vi "Get Ring Items.vi"(8 "error in (no error)":errorcluster, 11 "Scan Driver in":refnum<class "Scan Driver.lvclass">) -> (0 "error out":errorcluster, 1 "Reader":T2=enum."Photon Counter", 2 "Scanner":T1=enum."Magnetic Field", 3 "Scan Driver out":refnum<class "Scan Driver.lvclass">)   [LabVIEW 2012, in "Scan Driver.lvclass"]
doc: "If the object contains an \"XYZ.lvclass\", return the ring value for \"XYZ\". Class names must match the ring items exactly!"
uses:
  Scan Driver.lvclass
  Reader List.ctl
  Scanner List.ctl
  Scan Driver.lvclass/Scan Driver.ctl
  Readers/Reader/Reader.lvclass
panel:
  out "Reader name":string
  out "Scanner name":string
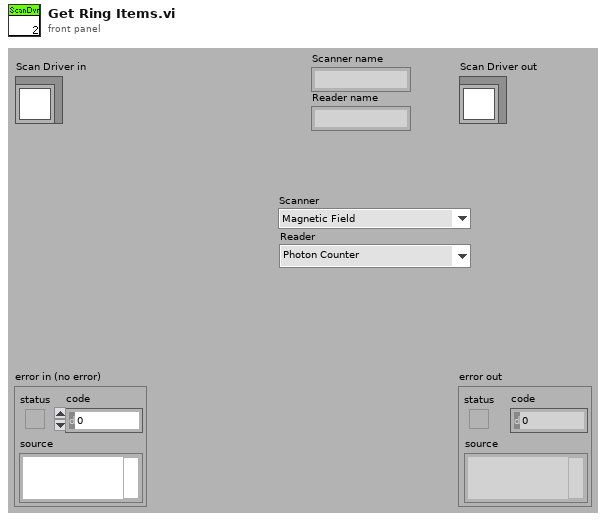
[diagram p1: front panel]
types:
  T1 = typedef "Scan Driver.lvclass/Scanner List.ctl" = enum16{"Analog Output Scan", "Continuous", "Dummy Scan", "Function Gen Scan", "Magnetic Field", "Magna Current Scan", "Magna Voltage Scan", "Microwave Freq Scan", "Pulse Gen Scan", "Pulse Gen Basic Scan", "Translation Stage Dual", "Wavelength", "Wavelength Digikröm", "Wavelength ActiveX", "Translation Stage Coarse", "Translation Stage Fine", "None"}
  T2 = typedef "Scan Driver.lvclass/Reader List.ctl" = enum16{"Anritsu Power Meter", "DAQmx Analog", "Dummy", "Lockin SR830", "Multimeter", "Photon Counter", "Power Meter", "Temperature Control"}
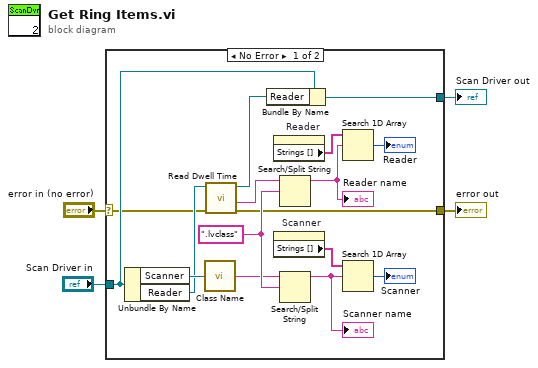
[diagram p0: block diagram]
diagram:
  n1 = case shown="No Error" "error in (no error)" {
    selector: "error in (no error)" -> [w12 w22]
    tunnel: [w11 w22] -> w3
    tunnel: [w14 w21] -> w1
    tunnel: "Scan Driver in" -> [w20 w21]
    frame No Error {
      w18 = ".lvclass" ("search string/char (-)")
      n2 = Unbundle By Name(w20) -> ("Scanner"=w19:refnum<class "Scanner.lvclass">, "Reader"=w16:refnum<class "Reader.lvclass">)
      n3 = call "Class Name.vi"("LabVIEW Object"=w19) -> ("Classname"=w17:string)
      n4 = call-dynamic "Read Dwell Time.vi"("error in (no error)"=w12, "Reader.lvclass in"=w16) -> ("error out"=w11:errorcluster, "Most Specific Classname"=w15:string, "Reader.lvclass out"=w13:refnum<class "Reader.lvclass">)  [unwired: 6 in, 1 out]
      n5 = Bundle By Name(cluster=w20, "Reader"=w13) -> (w14:refnum<class "Scan Driver.lvclass">)
      n6 = property on="Reader" class="Enum (strict)"() -> ("Strings []"=w10:string[])  [unwired: 2 in, 2 out]
      n7 = property on="Scanner" class="Enum (strict)"() -> ("Strings []"=w9:string[])  [unwired: 2 in, 2 out]
      n8 = Search/Split String(string=w15, search string/char (-)=w18) -> (substring before match=w6:string)  [unwired: 3 out]
      "Reader name" <- w6
      n9 = Search/Split String(string=w17, search string/char (-)=w18) -> (substring before match=w5:string)  [unwired: 3 out]
      "Scanner name" <- w5
      n10 = Search 1D Array(1D array=w10, element=w6) -> (index of element=→"Reader":i32)  [unwired: 1 out]
      n11 = Search 1D Array(1D array=w9, element=w5) -> (index of element=→"Scanner":i32)  [unwired: 1 out]
    }
    frame Error {
    }
  }
  "error out" <- w3
  "Scan Driver out" <- w1
